vi "VD-convertData.vi"(8 "error in (no error)":errorcluster, 10 "read buffer":T3 format="%x", 11 "VD-LV-LiteVNA in":refnum<class "VD-LV-LiteVNA.lvclass">) -> (0 "error out":errorcluster, 1 "Valid Data?":bool, 2 "VNA data":T1, 3 "VD-LV-LiteVNA out":refnum<class "VD-LV-LiteVNA.lvclass">, 4 "data status":T2)   [LabVIEW 2020, in "VD-LV-LiteVNA.lvclass"]
uses:
  VD-LV-LiteVNA.lvclass
  hardware-protocol/serial/HP-S-data.ctl
  VD-data_read_status.ctl
  VD-VNA_data.ctl
  VD-LV-data_format.ctl
  VD-LV-LiteVNA.lvclass/VD-LV-LiteVNA.ctl
  8b187b0d-c297-4cde-bfc3-90996bf8cc10.vi
  2a4fd52e-0b9b-40b6-a396-1a736fc8c1bc.vi
  hardware-protocol/serial/HP-S-Serial.lvclass
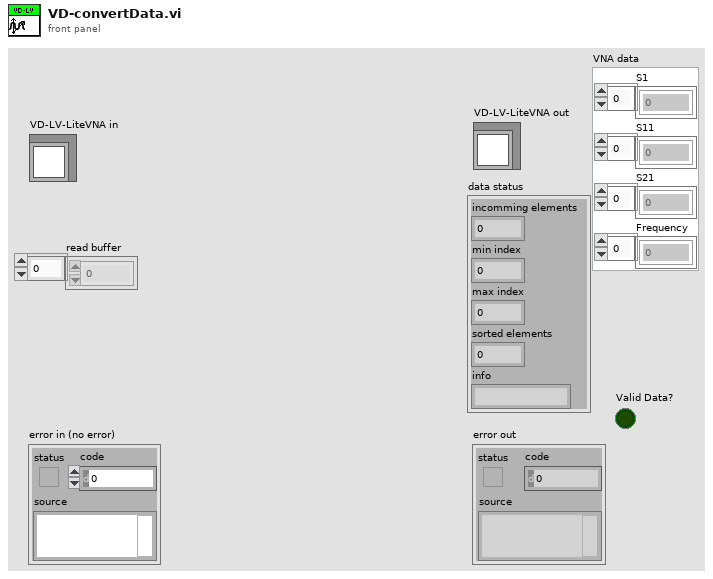
[diagram p1: front panel]
types:
  T1 = typedef "VD-LV-LiteVNA.lvclass/VD-VNA_data.ctl" = cluster{"S1":cdb[], "S11":cdb[], "S21":cdb[], "Frequency":u64[]}
  T2 = typedef "VD-LV-LiteVNA.lvclass/VD-data_read_status.ctl" = cluster{"incomming elements":i32, "min index":u16, "max index":u16, "sorted elements":i32, "info":string}
  T3 = typedef "HP-S-Serial.lvclass/HP-S-data.ctl" = u8[]
  T4 = typedef "VD-LV-LiteVNA.lvclass/VD-LV-data_format.ctl" = cluster{"OR":i32, "OI":i32, "RR":i32, "RI":i32, "IR":i32, "II":i32, "FREQ INDEX":u16, "reserved data":u32, "reserved data 2":u16}
  T5 = enum16{"big-endian, network order", "native, host order", "little-endian"}
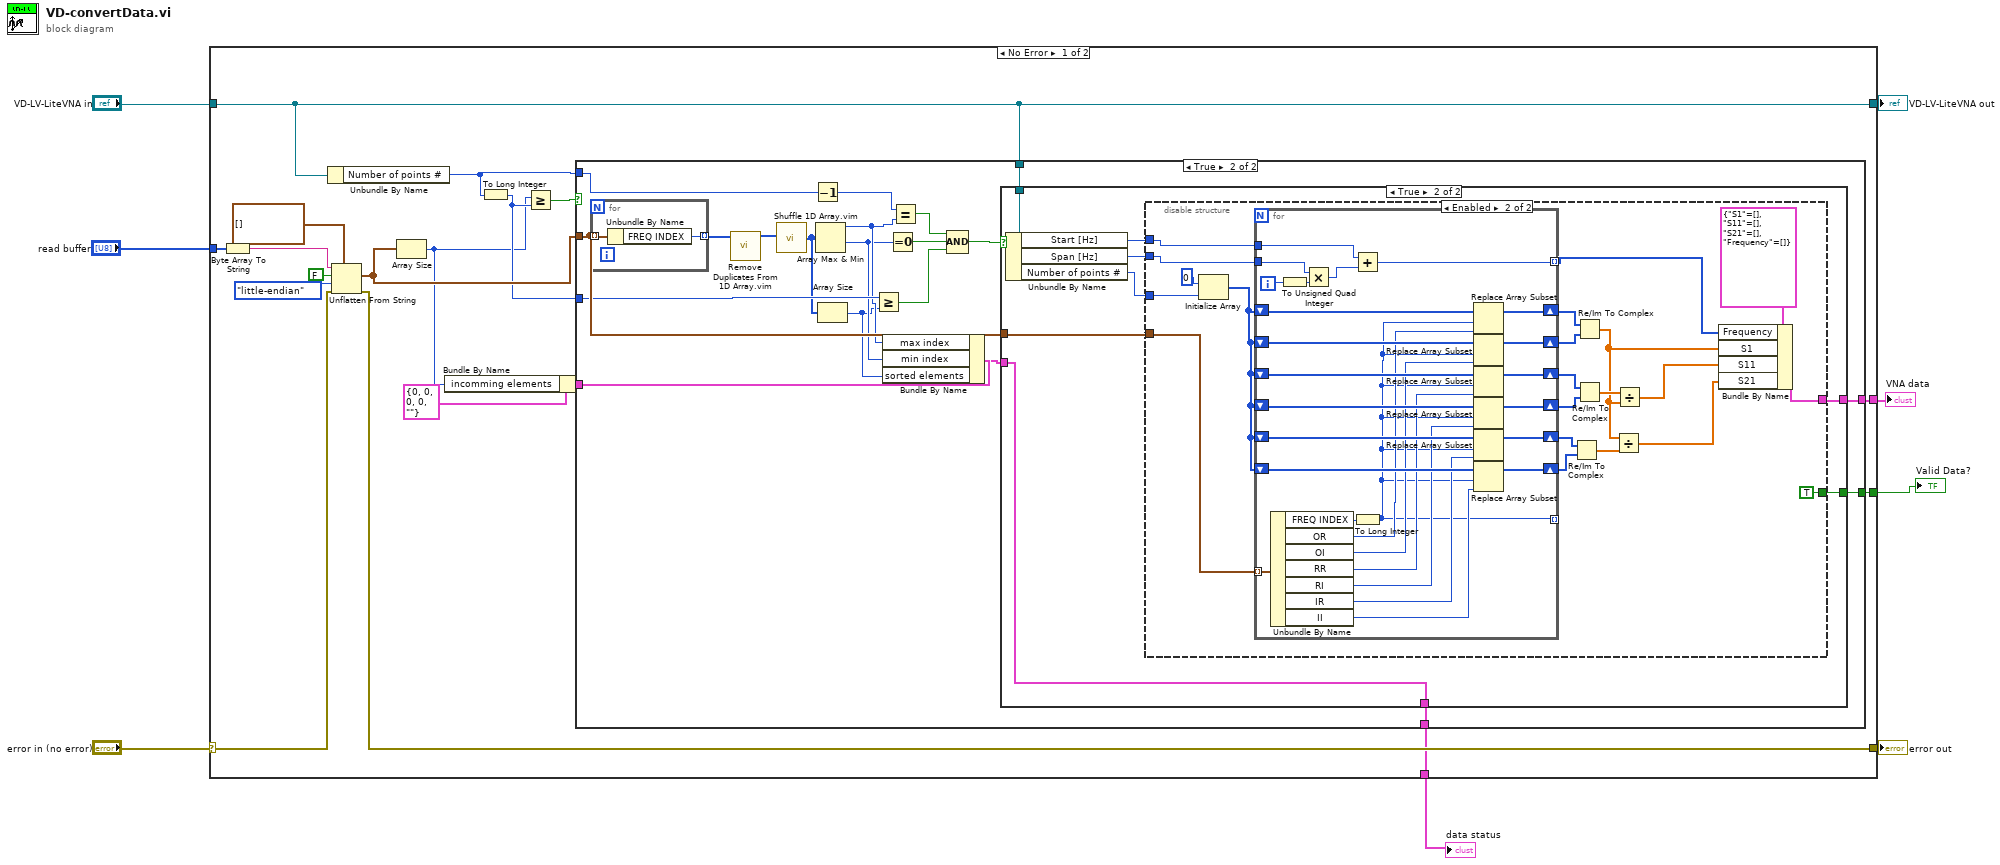
[diagram p0: block diagram]
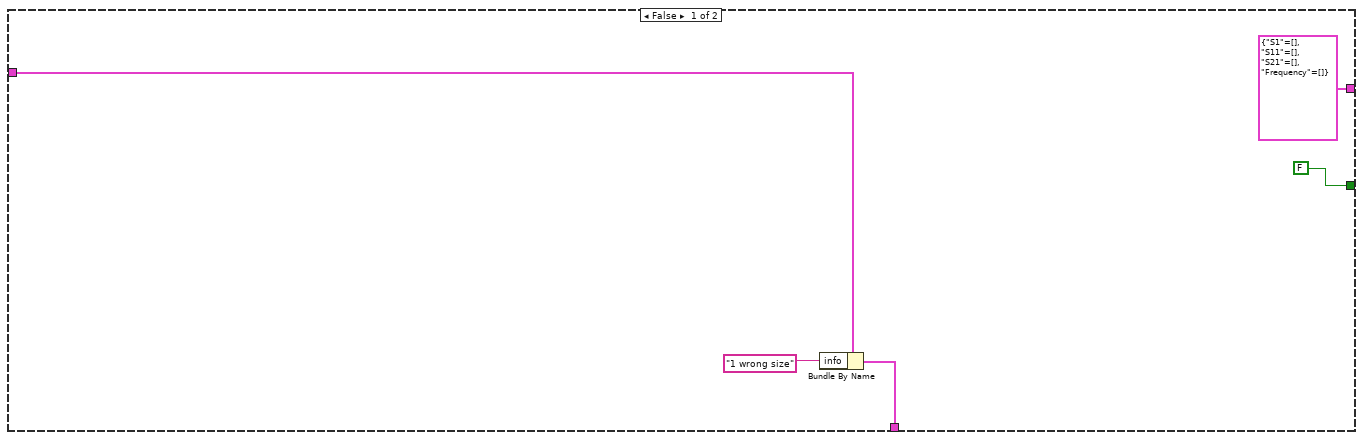
[diagram p2: hidden frame]
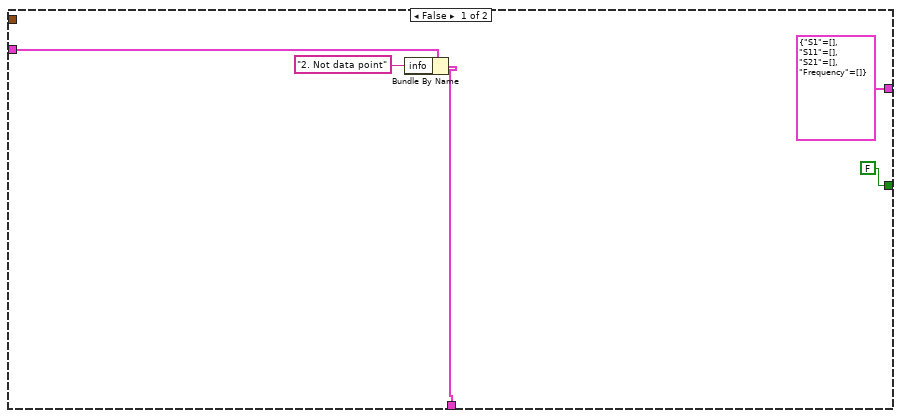
[diagram p3: hidden frame]
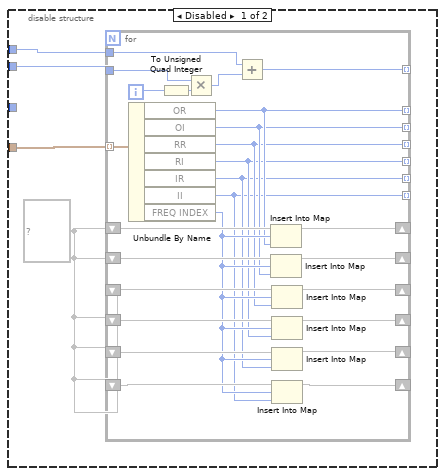
[diagram p4: hidden frame]
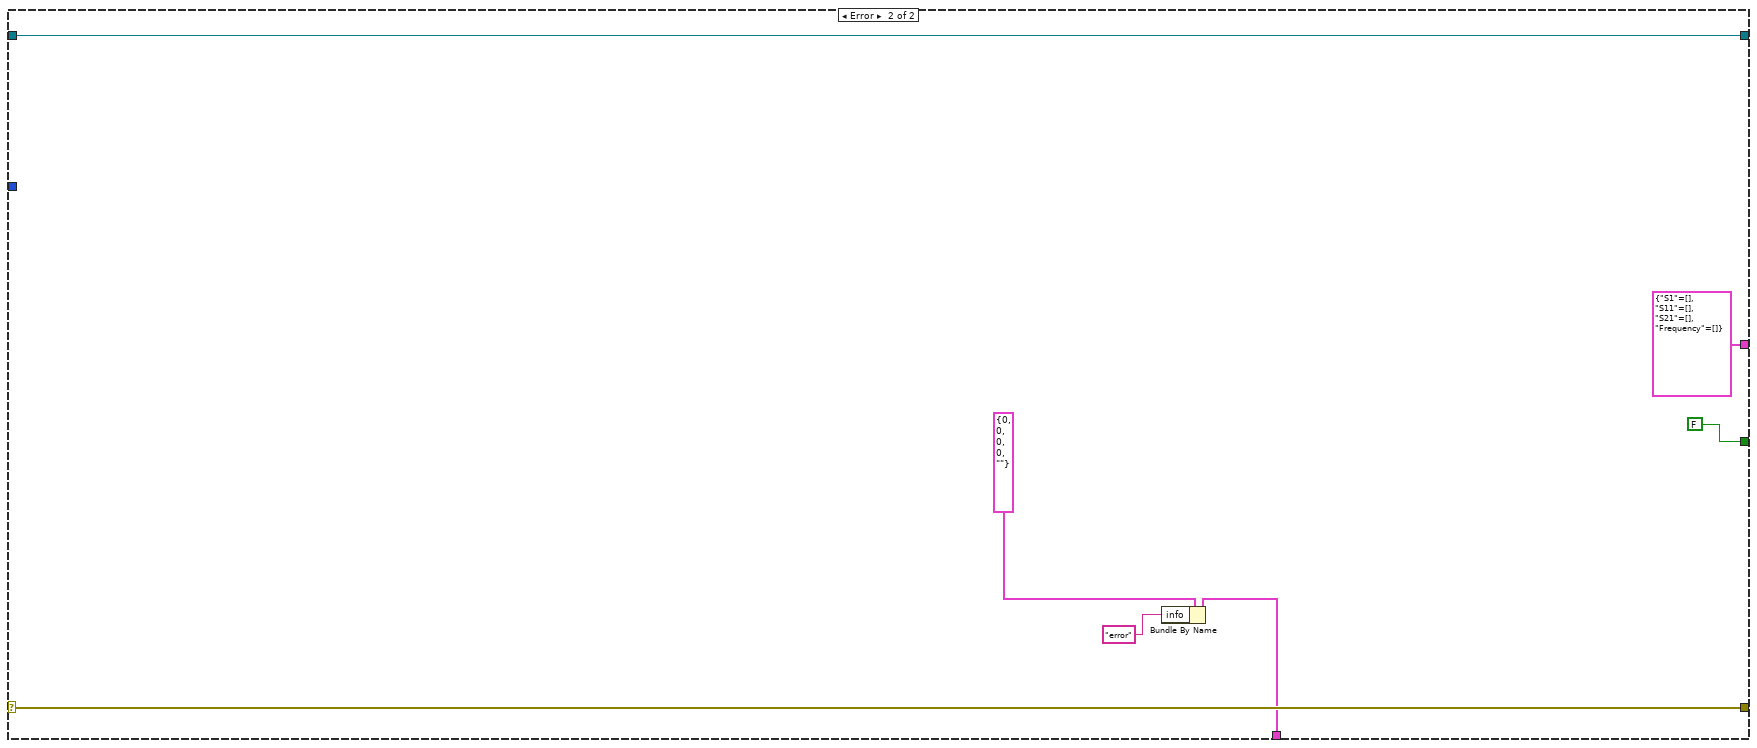
[diagram p5: hidden frame]
diagram:
  n1 = case shown="No Error" "error in (no error)" {
    selector: "error in (no error)" -> [w22 w151]
    tunnel: [w21 w151] -> w7
    tunnel: [w15 w150] -> w5
    tunnel: "VD-LV-LiteVNA in" -> [w15 w150]
    tunnel: "read buffer" -> [w23 _]
    tunnel: [w14 FALSE ("Valid Data?")] -> w3
    tunnel: [w10 w147] -> w2
    tunnel: [w9 T1 {"S1"=[], "S11"=[], "S21"=[], "Frequency"=[]} ("VNA data")] -> w1
    frame No Error {
      n2 = Byte Array To String(unsigned byte array=w23) -> (string=w24:string)
      n3 = Unbundle By Name(w15) -> ("Number of points #"=w17:u16)
      n4 = Unflatten From String(type=T4[] [] ("Array"), binary string=w24, data includes array or string size? (T)=FALSE, byte order (0:big-endian, network order)=T5."little-endian", error in (no error)=w22) -> (value=w19:T4[], error out=w21:errorcluster)  [unwired: 1 out]
      n5 = Array Size(array=w19) -> (size(s)=w11:i32)
      n6 = Bundle By Name(cluster=T2 {"incomming elements"=0, "min index"=0, "max index"=0, "sorted elements"=0, "info"=""} ("data status"), "incomming elements"=w11) -> (w12:T2)
      n7 = To Long Integer(number=w17) -> (32bit integer=w16:i32)
      n8 = Greater Or Equal?(x=w11, y=w16) -> (x >= y?=w18:bool)
      n9 = case shown="True" w18 {
        tunnel: w19 -> [_ w49]
        tunnel: w17 -> [_ w47]
        tunnel: w16 -> [_ w44]
        tunnel: w15 -> [_ w40]
        tunnel: [FALSE ("Valid Data?") w39] -> w14
        tunnel: w12 -> [w30 w38]
        tunnel: [w28 w33] -> w10
        tunnel: [T1 {"S1"=[], "S11"=[], "S21"=[], "Frequency"=[]} ("VNA data") w32] -> w9
        frame False {
          n10 = Bundle By Name(cluster=w30, "info"="1 wrong size" ("status")) -> (w28:T2)
        }
        frame True {
          n11 = for {
            tunnel: w49 -> [w144] mode=indexing
            tunnel: [w143] -> w51 mode=indexing
            n12 = Unbundle By Name(w144) -> ("FREQ INDEX"=w143:u16)
          }
          n13 = call "Remove Duplicates From 1D Array.vim"("array"=w51) -> ("array with duplicates removed"=w50:u16[])  [unwired: 10 in]
          n14 = call "Shuffle 1D Array.vim"("array"=w50) -> ("shuffled array"=w43:u16[])  [unwired: 4 in]
          n15 = Decrement(x=w47) -> (x-1=w48:u16)
          n16 = Array Max & Min(array=w43) -> (max value=w36:u16, min value=w35:u16)  [unwired: 2 out]
          n17 = Array Size(array=w43) -> (size(s)=w34:i32)
          n18 = Greater Or Equal?(x=w44, y=w34) -> (x >= y?=w42:bool)
          n19 = Bundle By Name(cluster=w38, "max index"=w36, "min index"=w35, "sorted elements"=w34) -> (w37:T2)
          n20 = Equal To 0?(x=w35) -> (x = 0?=w45:bool)
          n21 = Equal?(x=w48, y=w36) -> (x = y?=w46:bool)
          n22 = Compound Arithmetic op=AND(w46, w45, w42) -> (w41:bool)
          n23 = case shown="True" w41 {
            tunnel: w49 -> [_ w64]
            tunnel: w40 -> [_ w63]
            tunnel: [FALSE ("Valid Data?") w59] -> w39
            tunnel: w37 -> [w55 w58]
            tunnel: [w53 w58] -> w33
            tunnel: [T1 {"S1"=[], "S11"=[], "S21"=[], "Frequency"=[]} ("VNA data") w57] -> w32
            frame False {
              n24 = Bundle By Name(cluster=w55, "info"="2. Not data point" ("status")) -> (w53:T2)
            }
            frame True {
              n25 = Unbundle By Name(w63) -> ("Start [Hz]"=w62:u64, "Span [Hz]"=w61:u64, "Number of points #"=w60:u16)
              n26 = disable-structure shown="Enabled" {
                disable-tunnel: w64 -> [w67 w110]
                disable-tunnel: w62 -> [w66 w115]
                disable-tunnel: w61 -> [w65 w114]
                disable-tunnel: w60 -> [_ w112]
                disable-tunnel: [_ TRUE ("Valid Data?")] -> w59
                disable-tunnel: [_ w99] -> w57
                frame Disabled {
                  w68 = map{u16, i32} {} ("map")
                  n27 = for {
                    tunnel: w67 -> [w94] mode=indexing
                    tunnel: [w81] -> _ mode=indexing
                    tunnel: [w80] -> _ mode=indexing
                    tunnel: [w79] -> _ mode=indexing
                    tunnel: [w78] -> _ mode=indexing
                    tunnel: [w77] -> _ mode=indexing
                    tunnel: [w76] -> _ mode=indexing
                    shift-right: [w92] -> _
                    shift-left: w68 -> [w93]
                    shift-right: [w89] -> _
                    shift-left: w68 -> [w88]
                    shift-right: [w75] -> _
                    shift-left: w68 -> [w85]
                    shift-right: [w83] -> _
                    shift-left: w68 -> [w84]
                    shift-right: [w86] -> _
                    shift-left: w68 -> [w87]
                    shift-right: [w90] -> _
                    shift-left: w68 -> [w91]
                    tunnel: w66 -> [w71]
                    tunnel: w65 -> [w70]
                    tunnel: [w69] -> _ mode=indexing
                    i -> [w72]
                    n28 = Unbundle By Name(w94) -> ("OR"=w81:i32, "OI"=w80:i32, "RR"=w79:i32, "RI"=w78:i32, "IR"=w77:i32, "II"=w76:i32, "FREQ INDEX"=w82:u16)
                    n29 = To Unsigned Quad Integer(1:w72) -> (0:w74:u64)
                    n30 = Multiply(x=w70, y=w74) -> (x*y=w73:u64)
                    n31 = Add(x=w71, y=w73) -> (x+y=w69:u64)
                    n32 = Insert Into Map(map in=w93, key=w82, value=w81) -> (map out=w92:map{u16, i32})  [unwired: 2 out]
                    n33 = Insert Into Map(map in=w91, key=w82, value=w80) -> (map out=w90:map{u16, i32})  [unwired: 2 out]
                    n34 = Insert Into Map(map in=w88, key=w82, value=w79) -> (map out=w89:map{u16, i32})  [unwired: 2 out]
                    n35 = Insert Into Map(map in=w87, key=w82, value=w78) -> (map out=w86:map{u16, i32})  [unwired: 2 out]
                    n36 = Insert Into Map(map in=w85, key=w82, value=w77) -> (map out=w75:map{u16, i32})  [unwired: 2 out]
                    n37 = Insert Into Map(map in=w84, key=w82, value=w76) -> (map out=w83:map{u16, i32})  [unwired: 2 out]
                  }
                }
                frame Enabled {
                  n38 = Initialize Array(0, w112) -> (w111:i32[])
                  n39 = for {
                    tunnel: w110 -> [w142] mode=indexing
                    shift-right: [w130] -> w107
                    shift-left: w111 -> [w141]
                    shift-right: [w131] -> w106
                    shift-left: w111 -> [w140]
                    shift-right: [w132] -> w105
                    shift-left: w111 -> [w139]
                    shift-right: [w133] -> w104
                    shift-left: w111 -> [w138]
                    shift-right: [w134] -> w103
                    shift-left: w111 -> [w137]
                    shift-right: [w135] -> w102
                    shift-left: w111 -> [w136]
                    tunnel: w115 -> [w119]
                    tunnel: w114 -> [w121]
                    tunnel: [w117] -> w98 mode=indexing
                    tunnel: [w116] -> _ mode=indexing
                    i -> [w122]
                    n40 = Unbundle By Name(w142) -> ("FREQ INDEX"=w129:u16, "OR"=w128:i32, "OI"=w127:i32, "RR"=w126:i32, "RI"=w125:i32, "IR"=w124:i32, "II"=w123:i32)
                    n41 = To Unsigned Quad Integer(1:w122) -> (0:w120:u64)
                    n42 = Multiply(x=w121, y=w120) -> (x*y=w118:u64)
                    n43 = Add(x=w119, y=w118) -> (x+y=w117:u64)
                    n44 = To Long Integer(number=w129) -> (32bit integer=w116:i32)
                    n45 = Replace Array Subset(array=w141, new element=w128, index=w116) -> (w130:i32[])
                    n46 = Replace Array Subset(array=w140, new element=w127, index=w116) -> (w131:i32[])
                    n47 = Replace Array Subset(array=w139, new element=w126, index=w116) -> (w132:i32[])
                    n48 = Replace Array Subset(array=w138, new element=w125, index=w116) -> (w133:i32[])
                    n49 = Replace Array Subset(array=w137, new element=w124, index=w116) -> (w134:i32[])
                    n50 = Replace Array Subset(array=w136, new element=w123, index=w116) -> (w135:i32[])
                  }
                  n51 = Re/Im To Complex(1:w102, 2:w103) -> (0:w108:cdb[])
                  n52 = Re/Im To Complex(1:w106, 2:w107) -> (0:w97:cdb[])
                  n53 = Re/Im To Complex(1:w104, 2:w105) -> (0:w109:cdb[])
                  n54 = Divide(x=w108, y=w97) -> (x/y=w95:cdb[])
                  n55 = Divide(x=w109, y=w97) -> (x/y=w96:cdb[])
                  n56 = Bundle By Name(cluster=T1 {"S1"=[], "S11"=[], "S21"=[], "Frequency"=[]} ("VNA data"), "Frequency"=w98, "S1"=w97, "S11"=w96, "S21"=w95) -> (w99:T1)
                }
              }
            }
          }
        }
      }
    }
    frame Error {
      n57 = Bundle By Name(cluster=T2 {"incomming elements"=0, "min index"=0, "max index"=0, "sorted elements"=0, "info"=""} ("data status"), "info"="error" ("status")) -> (w147:T2)
    }
  }
  "error out" <- w7
  "VD-LV-LiteVNA out" <- w5
  "Valid Data?" <- w3
  "data status" <- w2
  "VNA data" <- w1
